vi "GlobalVar.vi"() -> ()   [LabVIEW 2015]
panel:
  out "License":string
  in  "UserGroup":string
  out "Language":u32
  in  "ConfigIniPath":path
  in  "LicensePath":path
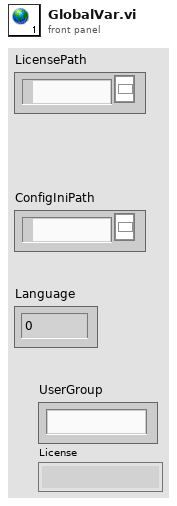
[diagram p1: front panel]
diagram:
